vi "CreateInitVI.vi"(4 "visitor class path":path, 5 "VariantAttNames":string[](array[string]), 6 "visitor base path":path, 7 "controls":cluster{"Style":u32, "Label.Text":string, i32}[](array[cluster]), 8 "error in (no error)":errorcluster, 11 "Class Reference":refnum<vi>) -> (0 "error out":errorcluster, 3 "dup Class Reference":refnum<vi>)   [LabVIEW 2009, in "HGF_VisitorGenerator.lvlib"]
doc: "create visitors override init.vi"
uses:
  HGF_VisitorGenerator.lvlib
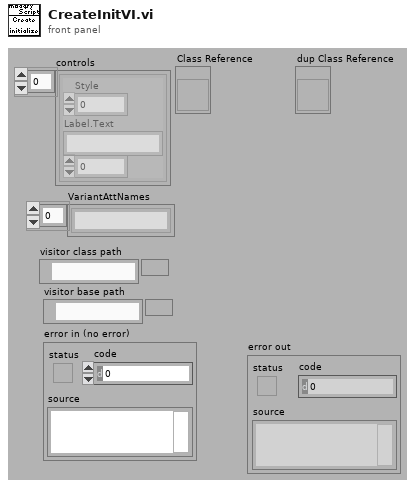
[diagram p1: front panel]
types:
  T1 = enum32{"invalid scope", "public", "private", "protected", "community"}
  T2 = enum32{"invalid VI type", "Standard VI", "Control VI", "Global VI", "Polymorphic VI", "Configuration VI", "SubSystem", "Facade VI", "Method VI", "Statechart Diagram VI"}
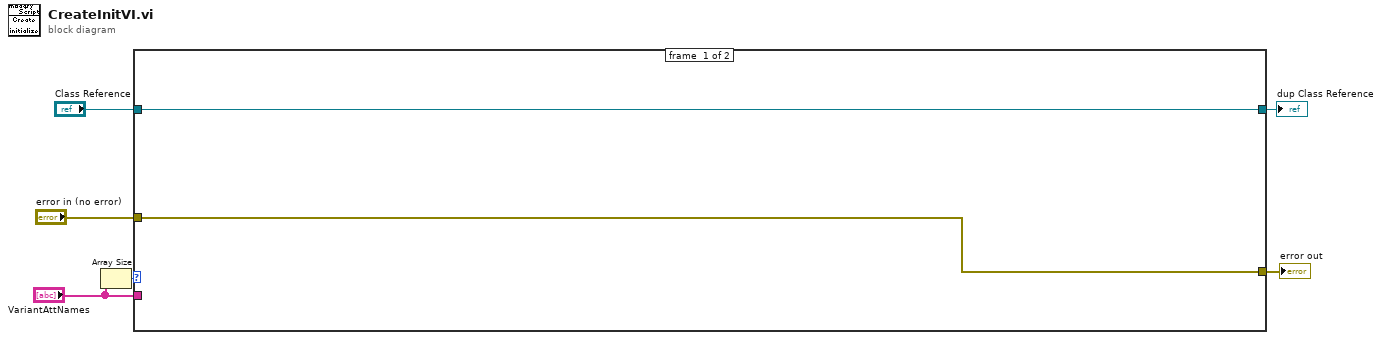
[diagram p0: block diagram]
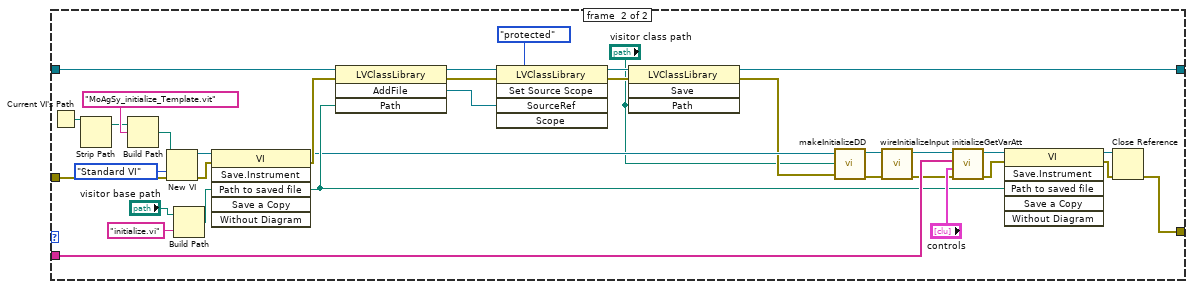
[diagram p2: hidden frame]
diagram:
  n1 = Array Size(array="VariantAttNames") -> (size(s)=w4:i32)
  n2 = case shown="Default" w4 {
    tunnel: "Class Reference" -> [w7 w41]
    tunnel: [w7 w42] -> w5
    tunnel: "error in (no error)" -> [w8 w38]
    tunnel: [w8 w27] -> w2
    tunnel: "VariantAttNames" -> [_ w32]
    frame #0 {
    }
    frame #1 {
      n3 = Current VI's Path() -> (path=w40:path)
      n4 = Strip Path(path=w40) -> (stripped path=w9:path)  [unwired: 1 out]
      n5 = Build Path(base path=w9, name or relative path="MoAgSy_initialize_Template.vit") -> (appended path=w11:path)
      n6 = New VI(8:w38, 9:T2."Standard VI" ("vi type (standard vi)"), 10:w11) -> (0:w34:errorcluster, 3:w37:refnum<vi>)  [unwired: 4 in]
      n7 = Build Path(base path="visitor base path", name or relative path="initialize.vi") -> (appended path=w30:path)
      n8 = invoke class="VI" method="Save.Instrument"(reference=w37, error in=w34, "Path to saved file"=w30) -> (reference out=w20:refnum<vi>, error out=w33:errorcluster)  [unwired: 3 in, 4 out]
      n9 = invoke class="LVClassLibrary" method="AddFile"(reference=w41, error in=w33, "Path"=w30) -> (reference out=w26:refnum<vi>, error out=w21:errorcluster, "AddFile"=w24:refnum<vi>)  [unwired: 1 in, 1 out]
      n10 = invoke class="LVClassLibrary" method="Set Source Scope"(reference=w26, error in=w21, "SourceRef"=w24, "Scope"=T1."protected" ("scope")) -> (reference out=w25:refnum<vi>, error out=w22:errorcluster)  [unwired: 1 in, 3 out]
      n11 = invoke class="LVClassLibrary" method="Save"(reference=w25, error in=w22, "Path"="visitor class path") -> (reference out=w42:refnum<vi>, error out=w14:errorcluster)  [unwired: 1 in, 2 out]
      n12 = call "makeInitializeDD.vi"("vi refnum"=w20, "Visitor class path"="visitor class path", "error in"=w14) -> ("vi refnum"=w17:refnum<vi>, "error out"=w19:errorcluster)  [unwired: 2 in]
      n13 = call "wireInitializeInput.vi"("error in (no error)"=w19, "vi refnum"=w17) -> ("error out"=w18:errorcluster, "dup vi refnum"=w16:refnum<vi>)  [unwired: 8 in]
      n14 = call "initializeGetVarAtt.vi"("error in"=w18, "controls"="controls", "VariantAttNames"=w32, "vi refnum"=w16) -> ("error out"=w12:errorcluster, "dup vi refnum"=w15:refnum<vi>)  [unwired: 2 in]
      n15 = invoke class="VI" method="Save.Instrument"(reference=w15, error in=w12, "Path to saved file"=w30) -> (reference out=w28:refnum<vi>, error out=w29:errorcluster)  [unwired: 3 in, 4 out]
      n16 = Close Reference(reference=w28, error in (no error)=w29) -> (error out=w27:errorcluster)
    }
  }
  "error out" <- w2
  "dup Class Reference" <- w5
